vi "Delta Time.vi"() -> ()   [LabVIEW 2022 SP3, in "Benchmark.lvlib"]
uses:
  Benchmark.lvlib
  8ca8b4a3-a15b-4534-87bf-3f66f767895e.vi
  <vilib>/Analysis/NI_AALBase.lvlib
panel:
  out "Std Dev":dbl format="%.1p"
  out "Mean":dbl format="%.1p"
  out "Histogram Graph":T1(graph)
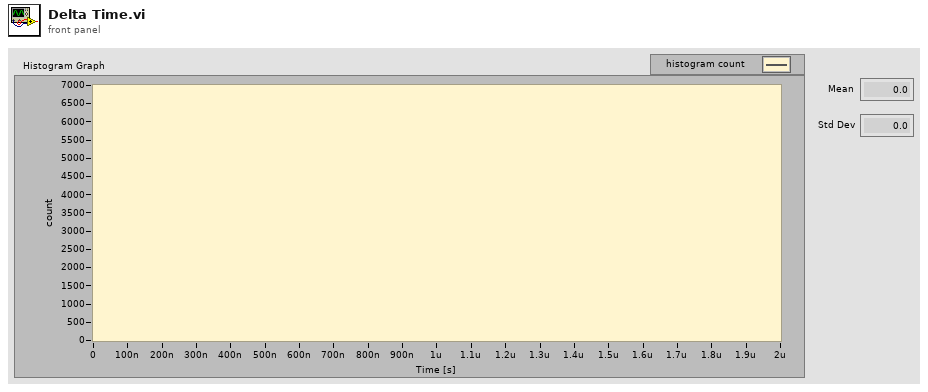
[diagram p1: front panel]
types:
  T1 = cluster{"X Values":dbl[], "Histogram: h(x)":i32[]}
  T2 = typedef "Core Data.ctl" = cluster{"Screen Dimensions":T3, "Camera":T4, "Transform":T5, "Line Colour":u32, "Fill Colour":u32, "Draw Lines":bool, "Projection Matrix":sgl[][], "Update Screen":bool, "Frame Buffer":refnum<data-value>, "Objects":T7[], "Camera Up":sgl, "Camera Left":sgl, "Camera Rotation":sgl, "Camera Forward":sgl, "Draw Triangles":bool, "Frame Buffer 2":refnum<data-value>, "Framebuffer":bool}
  T3 = typedef "Raster.lvlib/Screen Dimensions.ctl" = cluster{"Width":u32, "Height":u32}
  T4 = typedef "3D.lvlib/Camera.ctl" = cluster{"Field Of View":sgl, "Near Plane":sgl, "Far Plane":sgl}
  T5 = typedef "3D.lvlib/Transform.ctl" = cluster{"Position":T6, "Rotation":T6, "Scale":T6}
  T6 = typedef "3D.lvlib/Vector 3D.ctl" = cluster{"x":sgl, "y":sgl, "z":sgl}
  T7 = typedef "3D.lvlib/Mesh.ctl" = cluster{"Triangles":T8[]}
  T8 = typedef "3D.lvlib/Triangle 3D.ctl" = cluster{"Point 1":T6, "Point 2":T6, "Point 3":T6, "Fill Colour":u32}
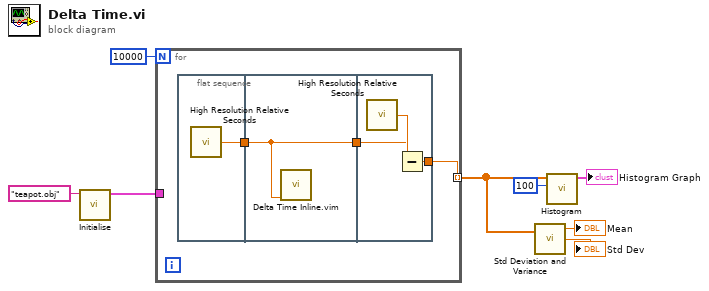
[diagram p0: block diagram]
diagram:
  n1 = call "Initialise.vi"("name or relative path"="teapot.obj") -> ("Core Data"=w5:T2)  [unwired: 9 in, 1 out]
  n2 = for {
    N: 10000 -> [_]
    tunnel: w5 -> [_]
    tunnel: [w9] -> w3 mode=indexing
    n3 = flat-sequence {
      tunnel: [w12] -> w11
      tunnel: w11 -> [w13]
      tunnel: [w13] -> w10
      tunnel: w10 -> [w15]
      tunnel: [w14] -> w9
      frame #0 {
        n4 = call <vilib>:"High Resolution Relative Seconds.vi"() -> ("relative seconds"=w12:dbl)
      }
      frame #1 {
        n5 = call "Delta Time Inline.vim"("value in"=w13) -> ()  [unwired: 8 in, 3 out]
      }
      frame #2 {
        n6 = call <vilib>:"High Resolution Relative Seconds.vi"() -> ("relative seconds"=w16:dbl)
        n7 = Subtract(x=w16, y=w15) -> (x-y=w14:dbl)
      }
    }
  }
  n8 = call <vilib>:"Std Deviation and Variance.vi"("X"=w3) -> ("mean"=→"Mean":dbl, "standard deviation"=→"Std Dev":dbl)  [unwired: 1 in, 1 out]
  n9 = call <vilib>:"Histogram.vi"("intervals"=100, "X"=w3) -> ("Histogram Graph"=→"Histogram Graph":T1)  [unwired: 6 in, 3 out]
